vi "Perform Action.vi"(8 "error in (no error)":errorcluster, 10 "Input":variant, 11 "DIO DAQmx PWM CFG in":refnum<class "CO DAQmx PWM CFG.lvclass">) -> (0 "error out":errorcluster, 2 "Output":variant, 3 "DIO DAQmx PWM CFG out":refnum<class "CO DAQmx PWM CFG.lvclass">)   [LabVIEW 2023, in "CO DAQmx PWM CFG.lvclass"]
uses:
  CO DAQmx PWM CFG.lvclass
  DAQmx/DAQmx Base CFG/DAQmx Base CFG.lvclass/DAQmx Base CFG.ctl
  Configuration/Configuration Semaphore/CFG Semaphore.lvclass/CFG Semaphore.ctl
  <vilib>/Utility/error.llb/Error Cluster From Error Code.vi
  <vilib>/ErrorRing/Error Ring.xnode
  CO DAQmx PWM CFG.lvclass/CO DAQmx PWM CFG.ctl
  DAQmx/DAQmx Base CFG/DAQmx Base CFG.lvclass
  <resource>/objmgr/daqmx.rc
  Configuration/Configuration Semaphore/CFG Semaphore.lvclass
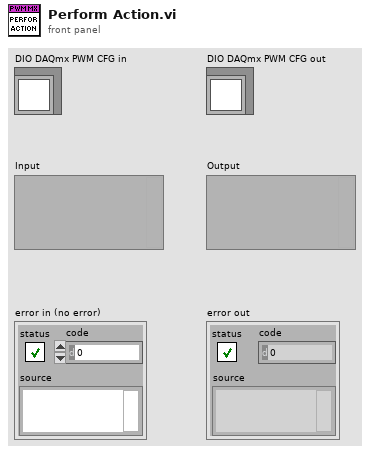
[diagram p1: front panel]
types:
  T1 = cluster{"Channel":string, "PWM Pams":cluster{"Frequency":dbl, "Duty Cycle":dbl}}
  T2 = typedef "Semaphore RefNum" = refnum<k1>
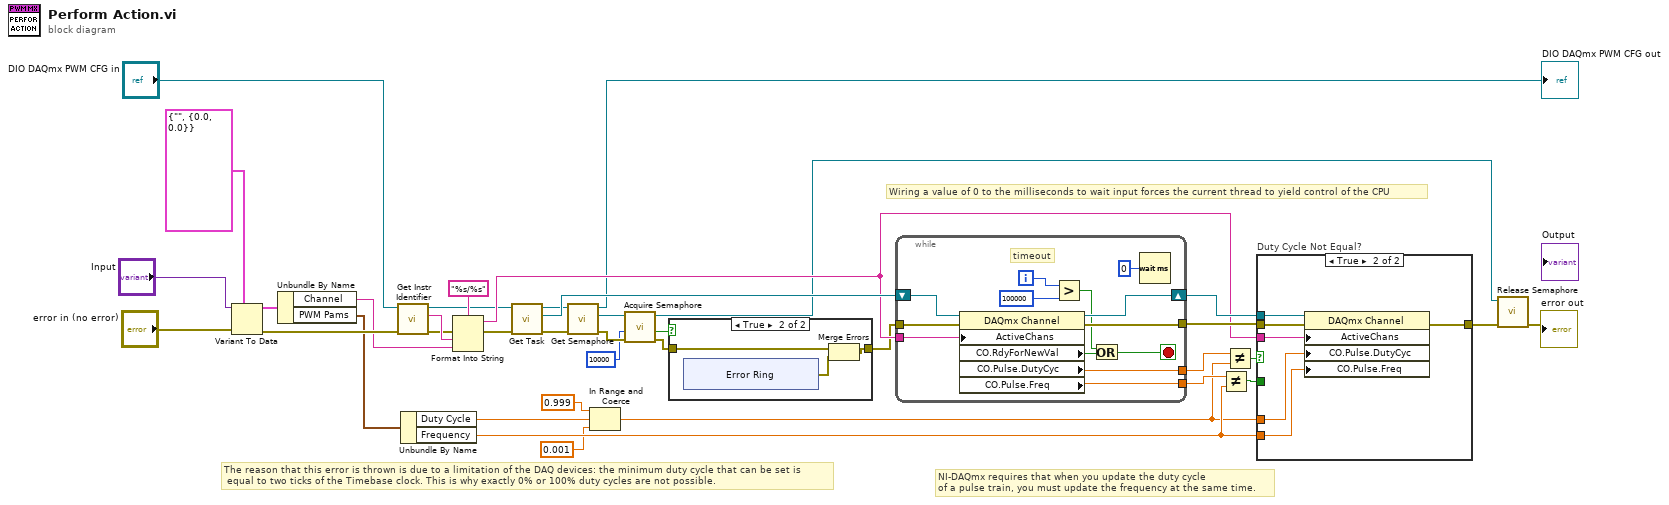
[diagram p0: block diagram]
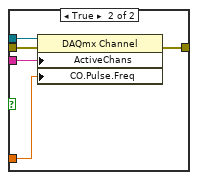
[diagram p4: hidden frame]
diagram:
  # "The reason that this error is thrown is due to a limitation of the DAQ devices: the minimum duty cycle that can be set is\n equal to two ticks of the Timebase clock. This is why exactly 0% or 100% duty cycles are not possible."
  # "Wiring a value of 0 to the milliseconds to wait input forces the current thread to yield control of the CPU"
  # "NI-DAQmx requires that when you update the duty cycle\nof a pulse train, you must update the frequency at the same time."
  n1 = Variant To Data(error in="error in (no error)", type=T1 {"Channel"="", "PWM Pams"={"Frequency"=0.0, "Duty Cycle"=0.0}}, Variant="Input") -> (data=w33:T1, error out=w34:errorcluster)
  n2 = Unbundle By Name(w33) -> ("Channel"=w28:string, "PWM Pams"=w26:cluster{"Frequency":dbl, "Duty Cycle":dbl})
  n3 = call-dynamic "Get Instr Identifier.vi"("error in (no error)"=w34, "Configuration Base in"="DIO DAQmx PWM CFG in") -> ("error out"=w27:errorcluster, "Instr Ident"=w29:string, "Configuration Base out"=w14:refnum<class "CO DAQmx PWM CFG.lvclass">)  [unwired: 7 in]
  n4 = Unbundle By Name(w26) -> ("Duty Cycle"=w24:dbl, "Frequency"=w20:dbl)
  n5 = Format Into String(format string="%s/%s", error in=w27, w29, w28) -> (resulting string=w16:string, error out=w1:errorcluster)  [unwired: 1 in]
  n6 = call "Get Task.vi"("DAQmx Base CFG in"=w14) -> ("Task"=w19:refnum<k21>, "DAQmx Base CFG out"=w15:refnum<class "CO DAQmx PWM CFG.lvclass">)  [unwired: 9 in]
  n7 = call "Get Semaphore.vi"("error in (no error)"=w1, "CFG Base in"=w15) -> ("error out"=w12:errorcluster, "Semaphore"=w13:T2, "CFG Base out"=→"DIO DAQmx PWM CFG out":refnum<class "CO DAQmx PWM CFG.lvclass">)  [unwired: 7 in]
  n8 = In Range and Coerce(upper limit=0.999, x=w24, lower limit=0.001) -> (coerced(x)=w4:dbl)  [unwired: 1 out]
  n9 = call <vilib>:"Acquire Semaphore.vi"("error in (no error)"=w12, "ms timeout (-1)"=10000, "semaphore"=w13) -> ("error out"=w6:errorcluster, "timed out"=w7:bool, "semaphore out"=w10:T2)  [unwired: 2 in]
  n10 = case shown="True" w7 {
    tunnel: w6 -> [w38 w40]
    tunnel: [w38 w39] -> w5
    frame False {
    }
    frame True {
      n11 = xnode "Error Ring"() -> ("error out"=w41:errorcluster)
      n12 = Merge Errors(w40, w41) -> (w39:errorcluster)
    }
  }
  n13 = while {
    tunnel: [w58] -> w23
    tunnel: w5 -> [w57]
    tunnel: [w55] -> w18
    tunnel: w16 -> [w54]
    shift-right: [w59] -> w25
    shift-left: w19 -> [w56]
    tunnel: [w48] -> w17
    i -> [w52]
    stop <- w50 stop-if-true
    # "timeout"
    n14 = property class="DAQmx Channel"(reference=w56, error in=w57, "ActiveChans"=w54) -> (reference out=w59:refnum<k21>, error out=w48:errorcluster, "CO.RdyForNewVal"=w53:bool, "CO.Pulse.DutyCyc"=w58:dbl, "CO.Pulse.Freq"=w55:dbl)
    n15 = Greater?(x=w52, y=100000) -> (0:w47:bool)
    n16 = Or(x=w47, y=w53) -> (x .or. y?=w50:bool)
    n17 = Wait (ms)(milliseconds to wait=u32 0) -> ()  [unwired: 1 out]
  }
  n18 = Not Equal?(x=w18, y=w20) -> (x != y?=w21:bool)
  n19 = Not Equal?(x=w23, y=w4) -> (x != y?=w22:bool)
  n20 = case "Duty Cycle Not Equal?" shown="True" w22 {
    tunnel: [w62 w77] -> w31
    tunnel: w20 -> [w63 w76]
    tunnel: w17 -> [w65 w75]
    tunnel: w25 -> [w61 w74]
    tunnel: w4 -> [_ w73]
    tunnel: w21 -> [w64 _]
    tunnel: w16 -> [w60 w72]
    frame False {
      n21 = case "Frequeny Not Equal?" shown="False" w64 {
        tunnel: w65 -> [w66 w71]
        tunnel: w63 -> [_ w68]
        tunnel: [w66 w70] -> w62
        tunnel: w61 -> [_ w69]
        tunnel: w60 -> [_ w67]
        frame False {
        }
        frame True {
          n22 = property class="DAQmx Channel"(reference=w69, error in=w71, "ActiveChans"=w67, "CO.Pulse.Freq"=w68) -> (error out=w70:errorcluster)  [unwired: 1 out]
        }
      }
    }
    frame True {
      n23 = property class="DAQmx Channel"(reference=w74, error in=w75, "ActiveChans"=w72, "CO.Pulse.DutyCyc"=w73, "CO.Pulse.Freq"=w76) -> (error out=w77:errorcluster)  [unwired: 1 out]
    }
  }
  n24 = call <vilib>:"Release Semaphore.vi"("error in (no error)"=w31, "semaphore"=w10) -> ("error out"=→"error out":errorcluster)  [unwired: 4 in, 1 out]
